vi "NI VeriStand - Run Workspace File.vi"(4 "Deploy System Definition (T)":bool=TRUE, 5 "Password (\"\") - DEPRECATED":string, 6 "Timeout (60000 ms)":u32=60000, 7 "User Name (\"\") - DEPRECATED":string, 8 "error in (no error)":errorcluster, 9 "Launch Workspace Window (F) - DEPRECATED":bool, 10 "System Definition File (.nivssdf)":path, 11 "WorkspaceManager in":T1) -> (0 "error out":errorcluster, 3 "WorkspaceManager out":T1)   [LabVIEW 2020, in "NI_VS Workspace ExecutionAPI.lvlib"]
doc: "Runs the workspace file you specify."
uses:
  <vilib>/NI VeriStand/Execution/Workspace/NI_VS Workspace ExecutionAPI.lvlib
  <vilib>/NI VeriStand/Execution/Workspace/WorkspaceAPI.ctl
  NationalInstruments.VeriStand.ClientAPI
panel:
  # "This VI has been deprecated in favor of NI VeriStand - Connect to System.vi. This VI no longer accepts a rig file path. Instead use a System Definition file path. The User Name, Password, and Launch Workspace Window inputs are deprecated."
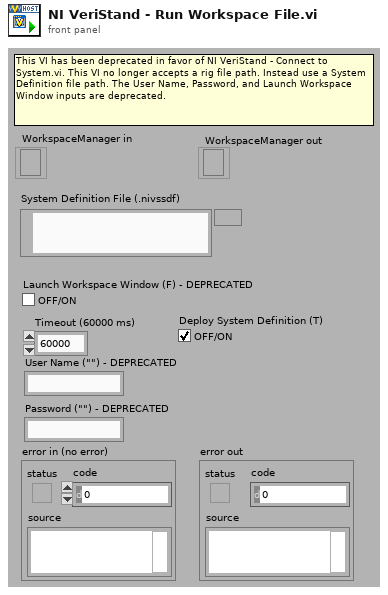
[diagram p1: front panel]
types:
  T1 = typedef "NI_VS Workspace ExecutionAPI.lvlib/WorkspaceAPI.ctl" = refnum<k24>
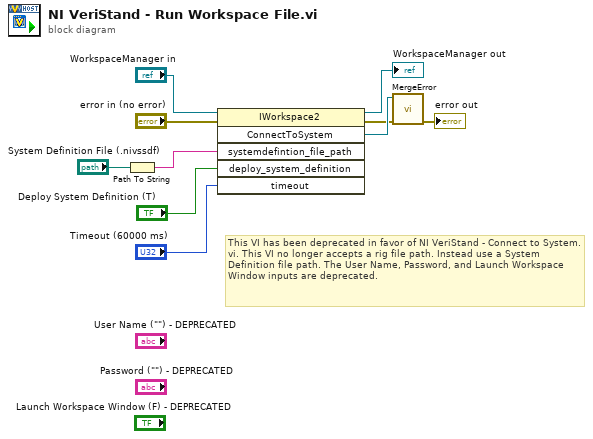
[diagram p0: block diagram]
diagram:
  # "This VI has been deprecated in favor of NI VeriStand - Connect to System.vi. This VI no longer accepts a rig file path. Instead use a System Definition file path. The User Name, Password, and Launch Workspace Window inputs are deprecated."
  n1 = Path To String(path="System Definition File (.nivssdf)") -> (string=w8:string)
  n2 = invoke class="IWorkspace2" method="ConnectToSystem"(reference="WorkspaceManager in", error in="error in (no error)", "systemdefintion_file_path"=w8, "deploy_system_definition"="Deploy System Definition (T)", "timeout"="Timeout (60000 ms)") -> (reference out=→"WorkspaceManager out":T1, error out=w4:errorcluster, "ConnectToSystem"=w5:refnum<k24>)  [unwired: 1 in, 3 out]
  n3 = call <vilib>:"MergeError.vi"("error in (no error)"=w4, "Error"=w5) -> ("error out"=→"error out":errorcluster)  [unwired: 9 out]
